vi "_builtins_icon_text.vi"(6 "Text Color (Black)":u32(colorbox), 8 "Justify (center)":enum8{"center", "left", "right"}(ring), 9 "Top (0)":i32, 10 "Text":string, 11 "Image in":T1) -> (3 "Image out":T1)   [LabVIEW 2019, in "Script.lvlib"]
doc: "Adds text to the <b>Image in</b> using the Small Fonts font. Escape characters included spaces (\"\\s\") and backslashes (\"\\\\\").\n\nCreated by: Ryan Pacini"
uses:
  Script.lvlib
  <vilib>/picture/picture.llb/imagedata.ctl
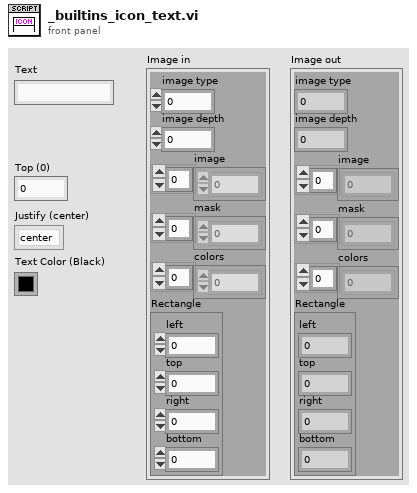
[diagram p1: front panel]
types:
  T1 = typedef "imagedata.ctl" = cluster{"image type":i32, "image depth":i32, "image":u8[], "mask":u8[], "colors":u32[], "Rectangle":cluster{"left":i16, "top":i16, "right":i16, "bottom":i16}}
  T2 = cluster{"left":i16, "top":i16, "right":i16, "bottom":i16}
  T3 = cluster{"left":i32, "top":i32, "right":i32, "bottom":i32}
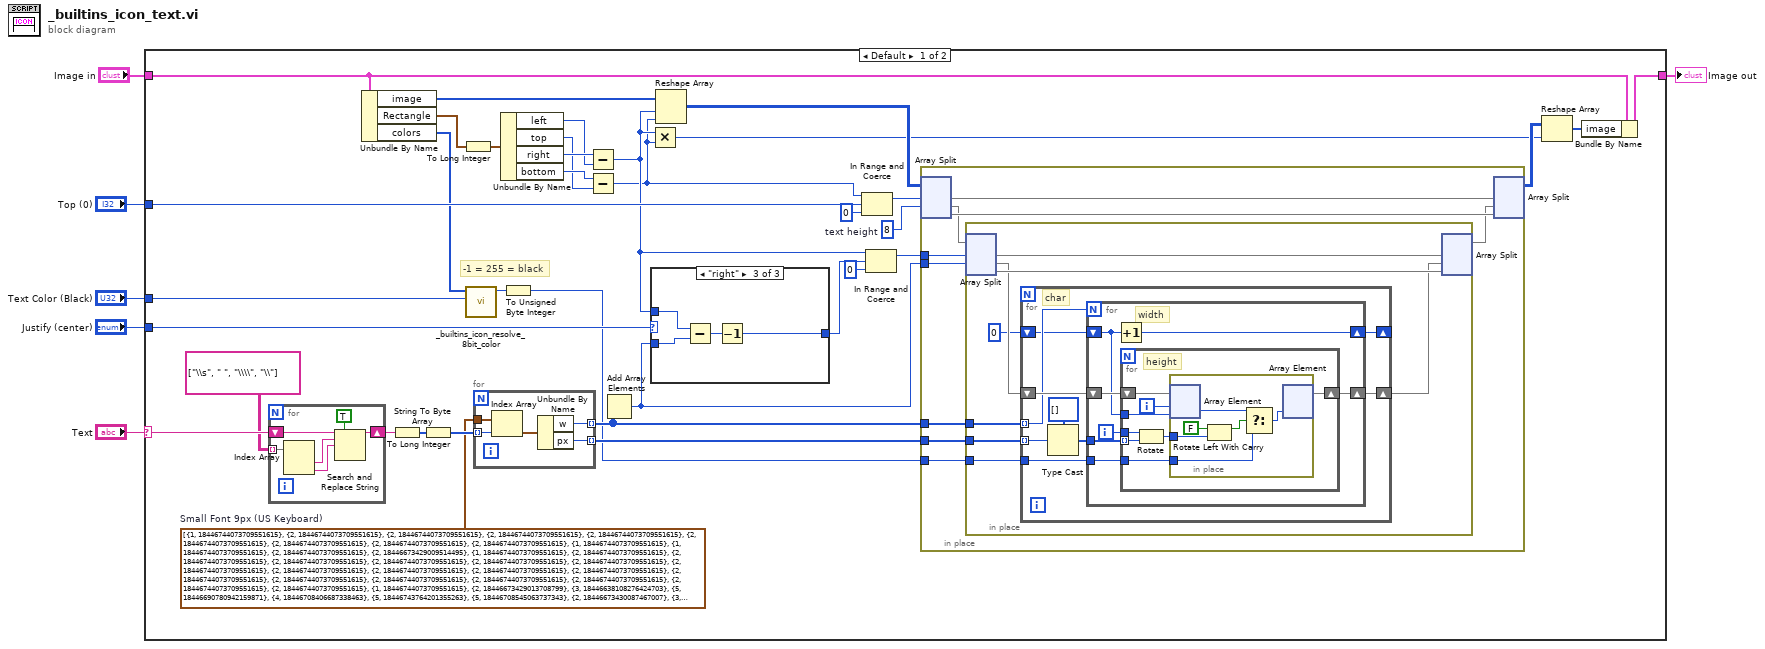
[diagram p0: block diagram]
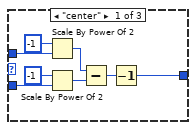
[diagram p2: hidden frame]
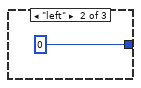
[diagram p3: hidden frame]
diagram:
  n1 = case shown="Default" "Text" {
    selector: "Text" -> [w29 _]
    tunnel: "Top (0)" -> [w35 _]
    tunnel: "Justify (center)" -> [w34 _]
    tunnel: "Text Color (Black)" -> [w8 _]
    tunnel: "Image in" -> [w14 w114]
    tunnel: [w12 w114] -> w1
    frame Default {
      w26 = cluster{"w":i32, "px":u64}[] [{"w"=1, "px"=18446744073709551615}, {"w"=2, "px"=18446744073709551615}, {"w"=2, "px"=18446744073709551615}, {"w"=2, "px"=18446744073709551615}, {"w"=2, "px"=18446744073709551615}, {"w"=2, "px"=18446744073709551615}, {"w"=2, "px"=18446744073709551615}, {"w"=2, "px"=18446744073709551615}, {"w"=2, "px"=18446744073709551615}, {"w"=1, "px"=18446744073709551615}, {"w"=1, "px"=18446744073709551615}, {"w"=2, "px"=18446744073709551615}, {"w"=2, "px"=18446673429009514495}, {"w"=1, "px"=18446744073709551615}, {"w"=2, "px"=18446744073709551615}, {"w"=2, "px"=18446744073709551615}, {"w"=2, "px"=18446744073709551615}, {"w"=2, "px"=18446744073709551615}, {"w"=2, "px"=18446744073709551615}, {"w"=2, "px"=18446744073709551615}, {"w"=2, "px"=18446744073709551615}, {"w"=2, "px"=18446744073709551615}, {"w"=2, "px"=18446744073709551615}, {"w"=2, "px"=18446744073709551615}, {"w"=2, "px"=18446744073709551615}, {"w"=2, "px"=18446744073709551615}, {"w"=2, "px"=18446744073709551615}, {"w"=2, "px"=18446744073709551615}, {"w"=2, "px"=18446744073709551615}, {"w"=2, "px"=18446744073709551615}, {"w"=2, "px"=18446744073709551615}, {"w"=2, "px"=18446744073709551615}, {"w"=1, "px"=18446744073709551615}, {"w"=2, "px"=18446673429013708799}, {"w"=3, "px"=18446638108276424703}, {"w"=5, "px"=18446690780942159871}, {"w"=4, "px"=18446708406687338463}, {"w"=5, "px"=18446743764201355263}, {"w"=5, "px"=18446708545063737343}, {"w"=2, "px"=18446673430087467007}, {"w"=3, "px"=18446708613381603295}, {"w"=3, "px"=18446673566987444159}, {"w"=3, "px"=18446638108276424703}, {"w"=4, "px"=18446743934389452799}, {"w"=2, "px"=18446744073709535167}, {"w"=3, "px"=18446744072098938879}, {"w"=2, "px"=18446744073709535231}, {"w"=3, "px"=18446708750283685887}, {"w"=4, "px"=18446708544392650751}, {"w"=3, "px"=18446708476481626111}, {"w"=4, "px"=18446638451332714495}, {"w"=4, "px"=18446638451335864319}, {"w"=4, "px"=18446726274015555583}, {"w"=4, "px"=18446620651649212415}, {"w"=4, "px"=18446708612843692031}, {"w"=4, "px"=18446620859148787711}, {"w"=4, "px"=18446708545197957119}, {"w"=4, "px"=18446708543859974143}, {"w"=2, "px"=18446744072635793407}, {"w"=2, "px"=18446744072635793343}, {"w"=3, "px"=18446744073168478207}, {"w"=3, "px"=18446744073703260159}, {"w"=3, "px"=18446744072633696255}, {"w"=3, "px"=18446673566452662271}, {"w"=7, "px"=18446717529295544295}, {"w"=5, "px"=18446691089777145855}, {"w"=5, "px"=18446620617285799935}, {"w"=5, "px"=18446690986835300351}, {"w"=5, "px"=18446620617956888575}, {"w"=4, "px"=18446620651914498047}, {"w"=4, "px"=18446620651914510335}, {"w"=5, "px"=18446682224699361279}, {"w"=5, "px"=18446664597616703487}, {"w"=2, "px"=18446673429009514495}, {"w"=4, "px"=18446726412530327551}, {"w"=5, "px"=18446664563659094015}, {"w"=4, "px"=18446673429009502207}, {"w"=6, "px"=18446668841648634879}, {"w"=5, "px"=18446664460714620927}, {"w"=5, "px"=18446690986701082623}, {"w"=5, "px"=18446620617286336511}, {"w"=5, "px"=18446690986700560383}, {"w"=5, "px"=18446620617285810175}, {"w"=5, "px"=18446682225374629887}, {"w"=4, "px"=18446620790429310975}, {"w"=5, "px"=18446664598422015999}, {"w"=4, "px"=18446655767837663231}, {"w"=6, "px"=18446668944729692159}, {"w"=4, "px"=18446655768639811583}, {"w"=4, "px"=18446655768642969599}, {"w"=4, "px"=18446620859146670079}, {"w"=3, "px"=18446638244637425567}, {"w"=3, "px"=18446673428474748927}, {"w"=3, "px"=18446638382615355295}, {"w"=4, "px"=18446708545740079103}, {"w"=4, "px"=18446744073709551375}, {"w"=3, "px"=18446673567526420479}, {"w"=4, "px"=18446744072898990079}, {"w"=4, "px"=18446673428471586815}, {"w"=4, "px"=18446744072900038655}, {"w"=4, "px"=18446726411993468927}, {"w"=4, "px"=18446744073167413247}, {"w"=3, "px"=18446708612844732415}, {"w"=4, "px"=18446744072898990063}, {"w"=4, "px"=18446673428471590911}, {"w"=2, "px"=18446673703887421439}, {"w"=2, "px"=18446673703887421375}, {"w"=4, "px"=18446673428738977791}, {"w"=2, "px"=18446673429009514495}, {"w"=6, "px"=18446744071690759167}, {"w"=4, "px"=18446744072093675519}, {"w"=4, "px"=18446744071825231871}, {"w"=4, "px"=18446744072093671359}, {"w"=4, "px"=18446744072898990063}, {"w"=3, "px"=18446744072094728191}, {"w"=3, "px"=18446744072094695423}, {"w"=3, "px"=18446743797216829439}, {"w"=4, "px"=18446744072362119167}, {"w"=4, "px"=18446744072362123263}, {"w"=5, "px"=18446744072496842751}, {"w"=4, "px"=18446744072365256703}, {"w"=4, "px"=18446744072365268927}, {"w"=4, "px"=18446744071828377599}, {"w"=3, "px"=18446708750820564959}, {"w"=2, "px"=18446673429009514495}, {"w"=3, "px"=18446673429548482495}, {"w"=4, "px"=18446690884834557951}, {"w"=2, "px"=18446673429009514495}, {"w"=2, "px"=18446673429009514495}, {"w"=0, "px"=18446744073709551615}, {"w"=2, "px"=18446744073709535167}, {"w"=4, "px"=18446691157831311295}, {"w"=3, "px"=18446744073709510495}, {"w"=5, "px"=18446744073709508607}, {"w"=4, "px"=18446708407762149343}, {"w"=4, "px"=18446708407762128863}, {"w"=4, "px"=18446708545740079103}, {"w"=6, "px"=18446699748771998719}, {"w"=5, "px"=15559874864230141951}, {"w"=3, "px"=18446744073168478207}, {"w"=6, "px"=18446607389188654079}, {"w"=0, "px"=18446744073709551615}, {"w"=2, "px"=18446673429009514495}, {"w"=0, "px"=18446744073709551615}, {"w"=0, "px"=18446744073709551615}, {"w"=2, "px"=18446673704965373951}, {"w"=2, "px"=18446673704965373951}, {"w"=3, "px"=18446638520593285119}, {"w"=3, "px"=18446638520593285119}, {"w"=3, "px"=18446744072092647423}, {"w"=4, "px"=18446744073702211583}, {"w"=6, "px"=18446744073701425151}, {"w"=4, "px"=18446690884834557951}, {"w"=6, "px"=18446475396326096895}, {"w"=3, "px"=18446568150234251263}, {"w"=3, "px"=18446744072633696255}, {"w"=6, "px"=18446744072764508159}, {"w"=0, "px"=18446744073709551615}, {"w"=2, "px"=18446673429009514495}, {"w"=4, "px"=12682048245608734719}, {"w"=1, "px"=18446744073709551615}, {"w"=2, "px"=18446743798827433919}, {"w"=4, "px"=18446744004180561887}, {"w"=4, "px"=18446726342203396095}, {"w"=4, "px"=18446655973998198783}, {"w"=4, "px"=18446655631198773247}, {"w"=2, "px"=18446673429009514431}, {"w"=4, "px"=18446690883489222559}, {"w"=3, "px"=18446638520593285119}, {"w"=5, "px"=18446690917446320127}, {"w"=2, "px"=18446673430087467007}, {"w"=3, "px"=18446744073168478207}, {"w"=4, "px"=18446744073702207487}, {"w"=2, "px"=18446744073705357311}, {"w"=5, "px"=18446690848995278847}, {"w"=4, "px"=18446480190918885375}, {"w"=2, "px"=18446743798831644671}, {"w"=3, "px"=18446744072092622847}, {"w"=2, "px"=18446673430087467007}, {"w"=2, "px"=18446743797757902847}, {"w"=2, "px"=18446673155209560063}, {"w"=4, "px"=18446744071014657919}, {"w"=3, "px"=18446743659779973087}, {"w"=2, "px"=18446744072635809791}, {"w"=2, "px"=18446744073709535039}, {"w"=2, "px"=18446743797757902847}, {"w"=2, "px"=18446743797757902847}, {"w"=3, "px"=18446744072633696255}, {"w"=5, "px"=18446743763127089151}, {"w"=5, "px"=18446743763127089151}, {"w"=5, "px"=18446743763127089151}, {"w"=3, "px"=18446743936268484575}, {"w"=4, "px"=18428694145881059327}, {"w"=4, "px"=18442204944763170815}, {"w"=4, "px"=18437701345135800319}, {"w"=4, "px"=18437701345135800319}, {"w"=4, "px"=18424190546253688831}, {"w"=4, "px"=18437701345135800319}, {"w"=6, "px"=18446713079674676223}, {"w"=5, "px"=18446690986835300335}, {"w"=4, "px"=18428606253136580607}, {"w"=4, "px"=18442117052018692095}, {"w"=4, "px"=18437613452391321599}, {"w"=4, "px"=18424102653509210111}, {"w"=2, "px"=18410644906868457471}, {"w"=3, "px"=18437666504632680447}, {"w"=3, "px"=18428553752261672959}, {"w"=3, "px"=18401707801479987199}, {"w"=4, "px"=18446638173500973055}, {"w"=5, "px"=18433153661832509439}, {"w"=5, "px"=18437683787446341631}, {"w"=5, "px"=18442187387073712127}, {"w"=5, "px"=18433180187818971135}, {"w"=5, "px"=18433180187818971135}, {"w"=5, "px"=18426424788377915391}, {"w"=4, "px"=18446743729570054143}, {"w"=5, "px"=18446682121349599231}, {"w"=5, "px"=18437657399167275007}, {"w"=5, "px"=18442160998794645503}, {"w"=5, "px"=18433153799539904511}, {"w"=5, "px"=18433153799539904511}, {"w"=4, "px"=18437648569388228607}, {"w"=4, "px"=18446673222579503103}, {"w"=4, "px"=18446708543855763455}, {"w"=4, "px"=18446708819807424511}, {"w"=4, "px"=18446726343273992191}, {"w"=4, "px"=18446691296340856831}, {"w"=4, "px"=18446691296340856831}, {"w"=4, "px"=18446656111968767999}, {"w"=4, "px"=18446708888526901247}, {"w"=6, "px"=18446744072764507135}, {"w"=4, "px"=18446744072900038639}, {"w"=4, "px"=18446673565910552575}, {"w"=4, "px"=18446708612843687935}, {"w"=4, "px"=18446708544124211199}, {"w"=4, "px"=18446656111163461631}, {"w"=2, "px"=18446603061339078655}, {"w"=3, "px"=18446708614455345151}, {"w"=3, "px"=18446673017766395903}, {"w"=3, "px"=18446743386510573567}, {"w"=3, "px"=18446743798288457727}, {"w"=4, "px"=18446638518977409023}, {"w"=4, "px"=18446673565642100735}, {"w"=4, "px"=18446726342200233983}, {"w"=4, "px"=18446708543855759359}, {"w"=4, "px"=18446691295267098623}, {"w"=4, "px"=18446656110895009791}, {"w"=4, "px"=18446744073165332479}, {"w"=4, "px"=18446744071823134719}, {"w"=4, "px"=18446673566178988031}, {"w"=4, "px"=18446726342737121279}, {"w"=4, "px"=18446708544392646655}, {"w"=4, "px"=18446656111431897087}, {"w"=4, "px"=18446726342740271039}, {"w"=4, "px"=18446673428471586751}, {"w"=4, "px"=18446656111435046847}]  # Small Font 9px (US Keyboard)
      w40 = 8  # text height
      # "-1 = 255 = black"
      n2 = for {
        shift-right: [w48] -> w30
        shift-left: w29 -> [w46]
        tunnel: string[][] [["\\s", " "], ["\\\\", "\\"]] ("escape chars (\\\\, \\s)") -> [w45] mode=indexing
        n3 = Index Array(array=w45) -> (element #1=w44:string, element #2=w43:string)  [unwired: 2 in]
        n4 = Search and Replace String(replace all?=TRUE ("replace all? (F)"), input string=w46, search string=w44, replace string=w43) -> (result string=w48:string)  [unwired: 4 in, 3 out]
      }
      n5 = Unbundle By Name(w14) -> ("image"=w24:u8[], "Rectangle"=w25:T2, "colors"=w9:u32[])
      n6 = String To Byte Array(string=w30) -> (unsigned byte array=w42:u8[])
      n7 = To Long Integer(number=w42) -> (32bit integer=w41:i32[])
      n8 = To Long Integer(number=w25) -> (32bit integer=w22:T3)
      n9 = call "_builtins_icon_resolve_8bit_color.vi"("color"=w8, "8-bit colors"=w9) -> ("index"=w7:i32)  [unwired: 8 in, 1 out]
      n10 = for {
        tunnel: w41 -> [w113] mode=indexing
        tunnel: w26 -> [w112]
        tunnel: [w110] -> w32 mode=indexing
        tunnel: [w109] -> w31 mode=indexing
        n11 = Index Array(array=w112, index=w113) -> (element=w111:cluster{"w":i32, "px":u64})
        n12 = Unbundle By Name(w111) -> ("w"=w110:i32, "px"=w109:u64)
      }
      n13 = Unbundle By Name(w22) -> ("left"=w20:i32, "top"=w18:i32, "right"=w21:i32, "bottom"=w19:i32)
      n14 = To Unsigned Byte Integer(number=w7) -> (unsigned 8bit integer=w27:u8)
      n15 = Subtract(x=w21, y=w20) -> (x-y=w11:i32)
      n16 = Subtract(x=w19, y=w18) -> (x-y=w10:i32)
      n17 = Add Array Elements(numeric array=w32) -> (sum=w28:i32)
      n18 = Multiply(x=w11, y=w10) -> (x*y=w15:i32)
      n19 = case shown="\"right\"" w34 {
        tunnel: w11 -> [w54 _ w61]
        tunnel: [w49 0 ("lower limit") w58] -> w33
        tunnel: w28 -> [w51 _ w59]
        frame "center" {
          n20 = Scale By Power Of 2(n=i16 -1, x=w54) -> (x*2^n=w53:i32)
          n21 = Scale By Power Of 2(n=i16 -1, x=w51) -> (x*2^n=w52:i32)
          n22 = Subtract(x=w53, y=w52) -> (x-y=w50:i32)
          n23 = Decrement(x=w50) -> (x-1=w49:i32)
        }
        frame "left" {
        }
        frame "right" {
          n24 = Subtract(x=w61, y=w59) -> (x-y=w60:i32)
          n25 = Decrement(x=w60) -> (x-1=w58:i32)
        }
      }
      n26 = Reshape Array(w24, w11, w10) -> (w23:u8[][])
      n27 = In Range and Coerce(upper limit=w10, x=w35, lower limit=0) -> (coerced(x)=w36:i32)  [unwired: 1 out]
      n28 = In Range and Coerce(upper limit=w11, x=w33, lower limit=0) -> (coerced(x)=w38:i32)  [unwired: 1 out]
      n29 = in-place {
        in-place-border: w38 -> [w67]
        in-place-border: w28 -> [w65]
        in-place-border: w32 -> [w64]
        in-place-border: w31 -> [w63]
        in-place-border: w27 -> [w62]
        n30 = in-place-split #1(w23, w36, w40) -> (w69:u8[][], w68:u8[][], w70:u8[][])
        n31 = in-place {
          in-place-border: w64 -> [w73]
          in-place-border: w63 -> [w75]
          in-place-border: w62 -> [w72]
          n32 = in-place-split #2(w68, w67, w65) -> (w78:u8[][], w76:u8[][], w77:u8[][])
          n33 = for {
            tunnel: w75 -> [w85] mode=indexing
            shift-right: [w86] -> w74
            shift-left: w76 -> [w87]
            tunnel: w73 -> [w82] mode=indexing
            tunnel: w72 -> [w81]
            shift-right: [w79] -> _
            shift-left: 0 -> [w80]
            # "char"
            n34 = Type Cast(type=u8[] [], x=w85) -> (*(type *) &x=w83:u8[])
            n35 = for {
              N: w82 -> [_]
              shift-right: [w93] -> w86
              shift-left: w87 -> [w94]
              tunnel: w83 -> [w92]
              shift-right: [w89] -> w79
              shift-left: w80 -> [w90]
              tunnel: w81 -> [w91]
              i -> [w88]
              # "width"
              n36 = Increment(x=w90) -> (x+1=w89:i32)
              n37 = for {
                shift-right: [w99] -> w93
                shift-left: w94 -> [w102]
                tunnel: w92 -> [w97] mode=indexing
                tunnel: w90 -> [w98]
                tunnel: w91 -> [w100]
                tunnel: w88 -> [w95]
                i -> [w101]
                # "height"
                n38 = Rotate(1:w97, 2:w95) -> (0:w96:u8)
                n39 = in-place {
                  in-place-border: w100 -> [w106]
                  in-place-border: w96 -> [w103]
                  n40 = in-place-array #3(w102, w101, w98) -> (w105:u8)
                  n41 = Rotate Left With Carry(2:w103, 3:FALSE ("carry")) -> (1:w107:bool)  [unwired: 1 out]
                  n42 = Select(t=w105, s=w107, f=w106) -> (s? t:f=w104:u8)
                  n43 = in-place-array #3(w104) -> (w99:u8[][])  [unwired: 2 out]
                }
              }
            }
          }
          n44 = in-place-split #2(w78, w74, w77) -> (w66:u8[][])  [unwired: 2 out]
        }
        n45 = in-place-split #1(w69, w66, w70) -> (w16:u8[][])  [unwired: 2 out]
      }
      n46 = Reshape Array(w16, w15) -> (w13:u8[])
      n47 = Bundle By Name(cluster=w14, "image"=w13) -> (w12:T1)
    }
    frame "" {
    }
  }
  "Image out" <- w1
